vi "ConfigurePath.vi"(8 "Error In":errorcluster, 10 "ConfigureName":string(combo)) -> (0 "Error Out":errorcluster, 1 "Folderpath":path, 2 "Filepath":path, 3 "file or folder exists?":bool)   [LabVIEW 2013]
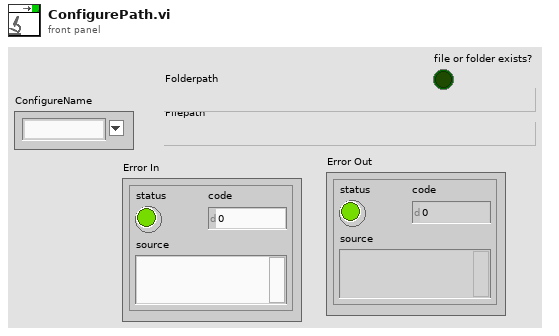
[diagram p1: front panel]
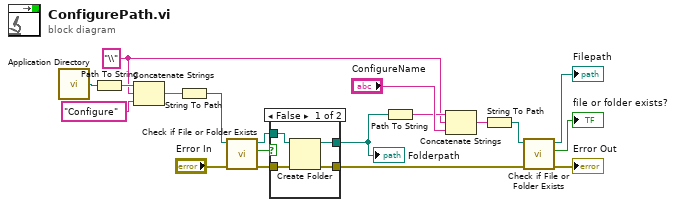
[diagram p0: block diagram]
diagram:
  w7 = "\\" ("string")
  n1 = call <vilib>:"Application Directory.vi"() -> ("Application Directory"=w19:path)
  n2 = Path To String(path=w19) -> (string=w18:string)
  n3 = Concatenate Strings(w18, w7, "Configure" ("string")) -> (w14:string)
  n4 = String To Path(string=w14) -> (path=w16:path)
  n5 = call <vilib>:"Check if File or Folder Exists.vi"("error in (no error)"="Error In", "path"=w16) -> ("error out"=w12:errorcluster, "file or folder exists?"=w15:bool, "dup path"=w13:path)  [unwired: 7 in]
  n6 = case shown="False" w15 {
    tunnel: [w21 w24] -> w4
    tunnel: [w20 w25] -> w5
    tunnel: w13 -> [w23 w25]
    tunnel: w12 -> [w22 w24]
    frame False {
      n7 = Create Folder(path (use dialog)=w23, error in=w22) -> (created path=w20:path, error out=w21:errorcluster)  [unwired: 1 in, 1 out]
    }
    frame True {
    }
  }
  "Folderpath" <- w5
  n8 = Path To String(path=w5) -> (string=w8:string)
  n9 = Concatenate Strings(w8, w7, "ConfigureName") -> (w11:string)
  n10 = String To Path(string=w11) -> (path=w10:path)
  n11 = call <vilib>:"Check if File or Folder Exists.vi"("error in (no error)"=w4, "path"=w10) -> ("error out"=→"Error Out":errorcluster, "file or folder exists?"=→"file or folder exists?":bool, "dup path"=→"Filepath":path)  [unwired: 7 in]
